vi "Request and Wait for Status.vi"(8 "error in (no error)":errorcluster) -> (0 "error out":errorcluster, 1 "timed out?":bool, 2 "Reply Payload":T1)   [LabVIEW 2015, in "Thermal Chamber Controller_DQMH.lvlib"]
doc: "Request the Thermal Chamber Controller to Update the Chamber Status and wait for the reply from the controller. Note that this is an example of a \"Request and Wait for Reply\" DQMH event.\n_____\nCreated using Delacor QMH Event Scripter 1.0.0.50.\n____\nDelacor QMH Thermal Chamber Examples 4.0.0.21\nCopyright (c) 2018, Delacor"
uses:
  Thermal Chamber Controller_DQMH.lvlib
  Request and Wait for Status (Reply Payload)--cluster.ctl
  Heater State--enum.ctl
  Request and Wait for Status Argument--cluster.ctl
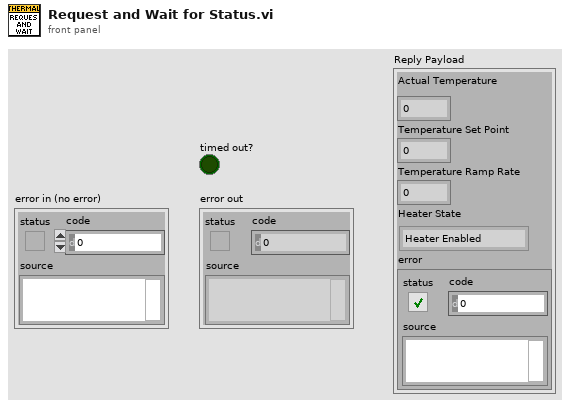
[diagram p1: front panel]
types:
  T1 = typedef "Thermal Chamber Controller_DQMH.lvlib/Request and Wait for Status (Reply Payload)--cluster.ctl" = cluster{"Actual Temperature":dbl, "Temperature Set Point":dbl, "Temperature Ramp Rate":dbl, "Heater State":T2, "error":errorcluster}
  T2 = typedef "Thermal Chamber Controller_DQMH.lvlib/Heater State--enum.ctl" = enum16{"Heater Enabled", "Heater Disabled"}
  T3 = typedef "Thermal Chamber Controller_DQMH.lvlib/Request and Wait for Status Argument--cluster.ctl" = cluster{"Wait Notifier":refnum<notifier>}
  T4 = typedef "Thermal Chamber Controller_DQMH.lvlib/Request Events--cluster.ctl" = cluster{"Stop Module":refnum<user-event>, "Show Panel":refnum<user-event>, "Hide Panel":refnum<user-event>, "Get Module Execution Status":refnum<user-event>, "Show Diagram":refnum<user-event>, "Update Set Point":refnum<user-event>, "Update Ramp Rate":refnum<user-event>, "Update Heater State":refnum<user-event>, "Update Chamber Status":refnum<user-event>, "Request and Wait for Status":refnum<user-event>}
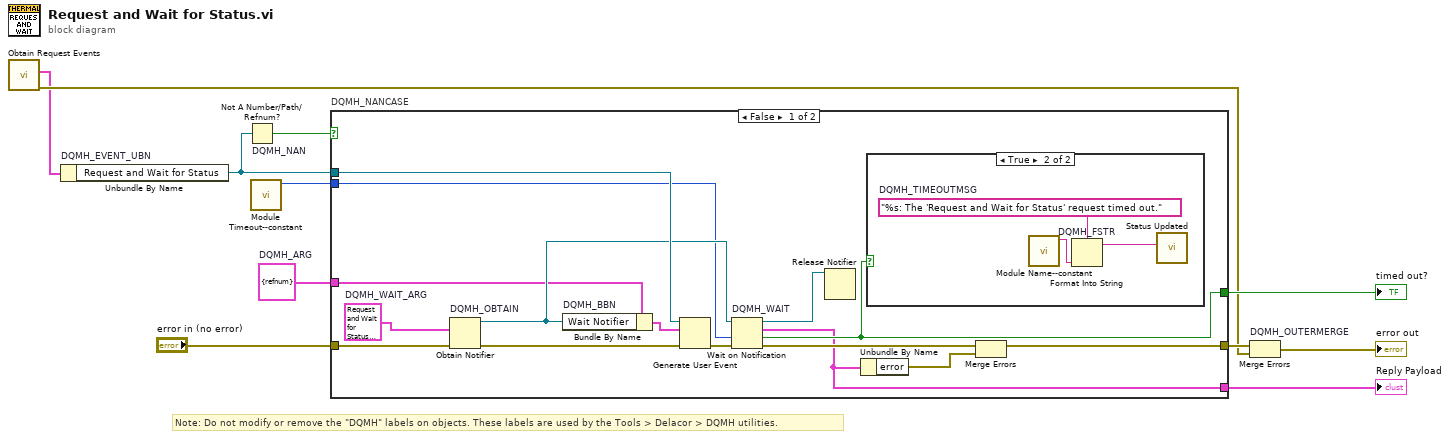
[diagram p0: block diagram]
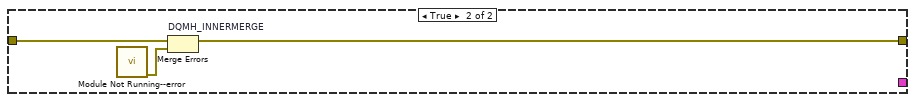
[diagram p3: hidden frame]
diagram:
  w5 = T3 {"Wait Notifier"=refnum}  # DQMH_ARG
  # "Note: Do not modify or remove the \"DQMH\" labels on objects. These labels are used by the Tools > Delacor > DQMH utilities."
  n1 = call "Obtain Request Events.vi"() -> ("error out"=w3:errorcluster, "Thermal Chamber Controller_DQMH Request Events"=w2:T4)  [unwired: 10 in]
  n2 = Unbundle By Name "DQMH_EVENT_UBN"(w2) -> ("Request and Wait for Status"=w8:refnum<user-event>)
  n3 = Not A Number/Path/Refnum? "DQMH_NAN"(number/path/refnum=w8) -> (NaN/Path/Refnum?=w7:bool)
  n4 = call "Module Timeout--constant.vi"() -> ("Module Timeout"=w4:i32)  [unwired: 11 in]
  n5 = case "DQMH_NANCASE" shown="False" w7 {
    tunnel: "error in (no error)" -> [w26 w32]
    tunnel: w8 -> [w24 _]
    tunnel: [w14 w31] -> w9
    tunnel: [w17 _] -> w6
    tunnel: w5 -> [w16 _]
    tunnel: w4 -> [w15 _]
    tunnel: [w13 _] -> w1
    frame False {
      w21 = T1 {"Actual Temperature"=0.0, "Temperature Set Point"=0.0, "Temperature Ramp Rate"=0.0, "Heater State"=enum."Heater Enabled", "error"={"status"=FALSE, "code"=0, "source"=""}}  # DQMH_WAIT_ARG
      n6 = Obtain Notifier "DQMH_OBTAIN"(notification data type=w21, error in (no error)=w26) -> (notifier out=w19:refnum<notifier>, error out=w22:errorcluster)  [unwired: 2 in, 1 out]
      n7 = Bundle By Name "DQMH_BBN"(cluster=w16, "Wait Notifier"=w19) -> (w23:T3)
      n8 = Generate User Event(user event=w24, event data cluster=w23, error in=w22) -> (error out=w25:errorcluster)  [unwired: 1 in, 1 out]
      n9 = Wait on Notification "DQMH_WAIT"(notifier=w19, timeout in ms (-1)=w15, error in (no error)=w25) -> (notifier out=w18:refnum<notifier>, notification=w13:T1, timed out?=w17:bool, error out=w20:errorcluster)  [unwired: 1 in]
      n10 = Release Notifier(notifier=w18) -> ()  [unwired: 2 in, 3 out]
      n11 = Unbundle By Name(w13) -> ("error"=w12:errorcluster)
      n12 = case shown="True" w17 {
        frame False {
        }
        frame True {
          w29 = "%s: The 'Request and Wait for Status' request timed out."  # DQMH_TIMEOUTMSG
          n13 = call "Module Name--constant.vi"() -> ("Module Name"=w28:string)  [unwired: 11 in]
          n14 = Format Into String "DQMH_FSTR"(format string=w29, w28) -> (resulting string=w27:string)  [unwired: 2 in, 1 out]
          n15 = call "Status Updated.vi"("Status"=w27) -> ()  [unwired: 10 in, 1 out]
        }
      }
      n16 = Merge Errors(w20, w12) -> (w14:errorcluster)
    }
    frame True {
      n17 = call "Module Not Running--error.vi"() -> ("error out"=w30:errorcluster)  [unwired: 11 in]
      n18 = Merge Errors "DQMH_INNERMERGE"(w32, w30) -> (w31:errorcluster)
    }
  }
  "timed out?" <- w6
  "Reply Payload" <- w1
  n19 = Merge Errors "DQMH_OUTERMERGE"(w9, w3) -> (→"error out":errorcluster)
